vi "LSI218Data_initialize.vi"(4 "LSI218Settings(A-F)":T2(array[cluster])=[{"LSIName"="LSI218A", "Labels"=["N.C.", "N.C.", "N.C.", "N.C.", "N.C.", "N.C.", "N.C.", "N.C."], "SensorLocations"=[enum."N.C.", enum."N.C.", enum."N.C.", enum."N.C.", enum."N.C.", enum."N.C.", enum."N.C.", enum."N.C."], "Active?"=FALSE, "VISA res. name"=""}, {"LSIName"="LSI218B", "Labels"=["N.C.", "N.C.", "N.C.", "N.C.", "N.C.", "N.C.", "N.C.", "N.C."], "SensorLocations"=[enum."N.C.", enum."N.C.", enum."N.C.", enum."N.C.", enum."N.C.", enum."N.C.", enum."N.C.", enum."N.C."], "Active?"=FALSE, "VISA res. name"=""}, {"LSIName"="LSI218C", "Labels"=["N.C.", "N.C.", "N.C.", "N.C.", "N.C.", "N.C.", "N.C.", "N.C."], "SensorLocations"=[enum."N.C.", enum."N.C.", enum."N.C.", enum."N.C.", enum."N.C.", enum."N.C.", enum."N.C.", enum."N.C."], "Active?"=FALSE, "VISA res. name"=""}, {"LSIName"="LSI218D", "Labels"=["N.C.", "N.C.", "N.C.", "N.C.", "N.C.", "N.C.", "N.C.", "N.C."], "SensorLocations"=[enum."N.C.", enum."N.C.", enum."N.C.", enum."N.C.", enum."N.C.", enum."N.C.", enum."N.C.", enum."N.C."], "Active?"=FALSE, "VISA res. name"=""}, {"LSIName"="LSI218E", "Labels"=["N.C.", "N.C.", "N.C.", "N.C.", "N.C.", "N.C.", "N.C.", "N.C."], "SensorLocations"=[enum."N.C.", enum."N.C.", enum."N.C.", enum."N.C.", enum."N.C.", enum."N.C.", enum."N.C.", enum."N.C."], "Active?"=FALSE, "VISA res. name"=""}, {"LSIName"="LSI218F", "Labels"=["N.C.", "N.C.", "N.C.", "N.C.", "N.C.", "N.C.", "N.C.", "N.C."], "SensorLocations"=[enum."N.C.", enum."N.C.", enum."N.C.", enum."N.C.", enum."N.C.", enum."N.C.", enum."N.C.", enum."N.C."], "Active?"=FALSE, "VISA res. name"=""}], 5 "FileFormat":string, 7 "base path":path, 8 "error in (no error)":errorcluster, 9 "InstName":string, 10 "RunIdentifier":string, 11 "LSI218Data in":refnum<class "LSI218Data.lvclass">) -> (0 "error out":errorcluster, 1 "Status":T1(ring), 2 "AllLabels":string[](array[string]), 3 "LSI218Data out":refnum<class "LSI218Data.lvclass">)   [LabVIEW 2020, in "LSI218Data.lvclass"]
uses:
  LSI218Data.lvclass
  LSI218Data.lvclass/LSI218Data.ctl
  istr.lib/Lake Shore Cryotronics 218/Lake Shore Cryotronics 218.lvlib
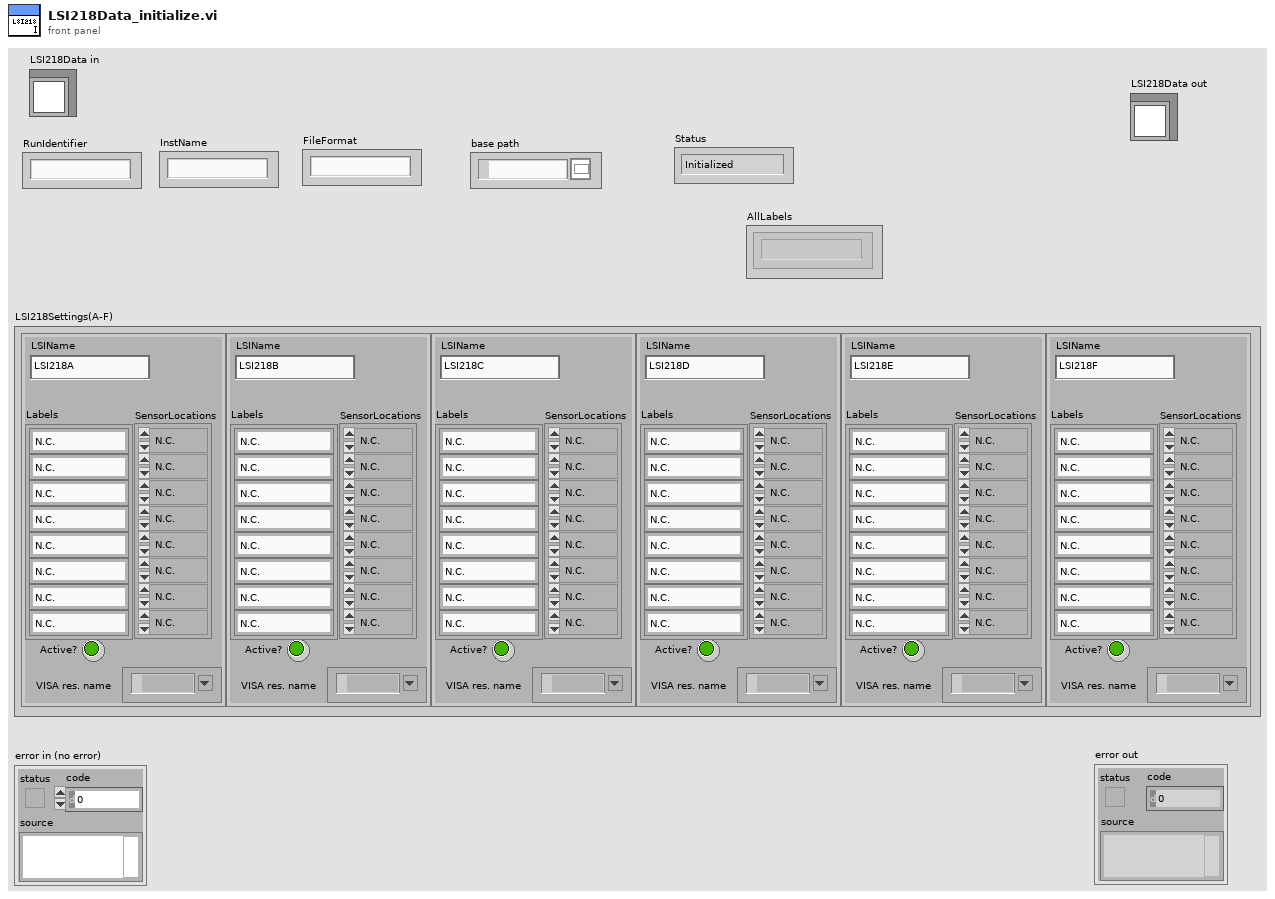
[diagram p1: front panel]
types:
  T1 = enum16{"Initialized", "Ready", "Measuring", "Terminated"}
  T2 = cluster{"LSIName":string, "Labels":string[], "SensorLocations":enum16{"N.C.", "T3He1-1", "T3He1-2", "T3He1-3", "T3He1-4", "T3He2-1", "T3He2-2", "T3He3", "T3He4", "T3He5", "T3He6-1", "T3He6-2", "T3He7-1", "T3He7-2", "T3He8", "T3He9", "T3He10", "T4He1", "T4He2-1", "T4He2-2", "T4He3-1", "T4He3-2", "T4He3-3", "T4He3-4", "T4He4", "T4He5", "T4He6", "T4He7", "T4He8", "T4He9", "T4He10", "T1K1", "T1K2", "T1K3-1", "T1K3-2", "T1K4", "T1K5", "T1K6", "TIP1", "TIP2", "TIP3", "TIP4", "TIP5", "TIP6", "TIP7", "TTH1", "TTH2", "TTH3", "TTH4"}[], "Active?":bool, "VISA res. name":refnum<visa-resource-name>}[]
  T3 = enum16{"open", "replace", "create", "open or create", "replace or create", "replace or create with confirmation"}
  T4 = cluster{"LSIName":string, "Labels":string[], "SensorLocations":enum16{"N.C.", "T3He1-1", "T3He1-2", "T3He1-3", "T3He1-4", "T3He2-1", "T3He2-2", "T3He3", "T3He4", "T3He5", "T3He6-1", "T3He6-2", "T3He7-1", "T3He7-2", "T3He8", "T3He9", "T3He10", "T4He1", "T4He2-1", "T4He2-2", "T4He3-1", "T4He3-2", "T4He3-3", "T4He3-4", "T4He4", "T4He5", "T4He6", "T4He7", "T4He8", "T4He9", "T4He10", "T1K1", "T1K2", "T1K3-1", "T1K3-2", "T1K4", "T1K5", "T1K6", "TIP1", "TIP2", "TIP3", "TIP4", "TIP5", "TIP6", "TIP7", "TTH1", "TTH2", "TTH3", "TTH4"}[], "Active?":bool, "VISA res. name":refnum<visa-resource-name>}
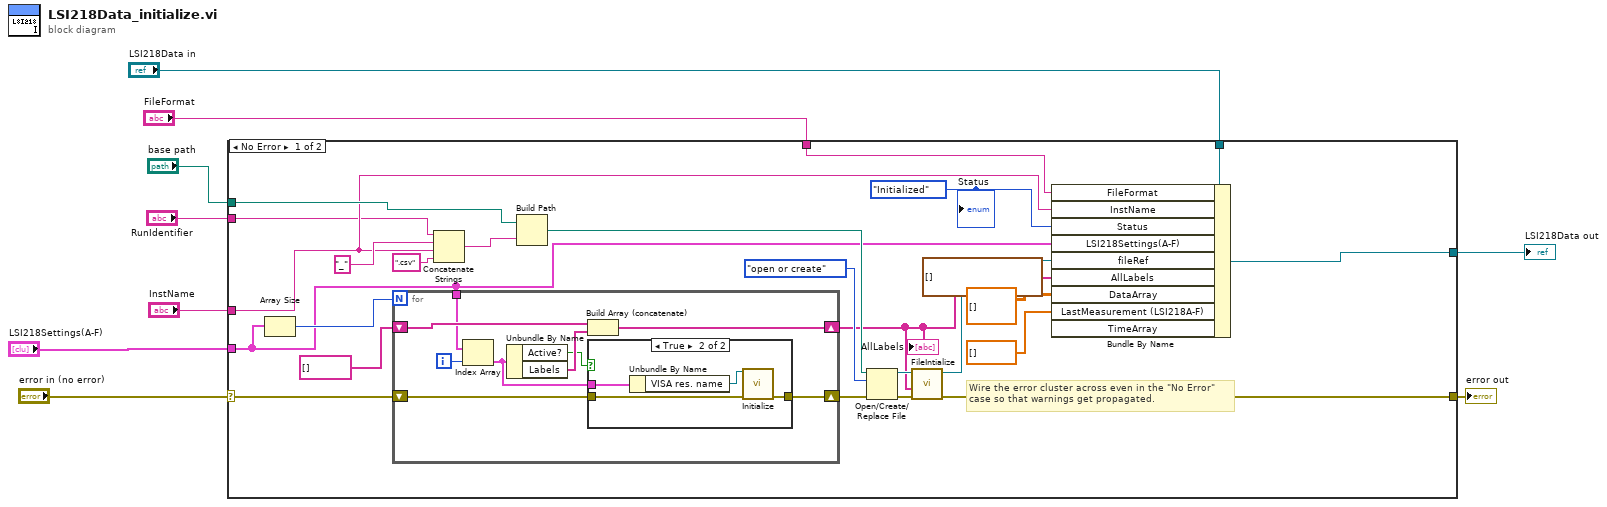
[diagram p0: block diagram]
diagram:
  n1 = case shown="No Error" "error in (no error)" {
    selector: "error in (no error)" -> [w17 w50]
    tunnel: [w16 w50] -> w8
    tunnel: [w33 w49] -> w1
    tunnel: "LSI218Settings(A-F)" -> [w12 _]
    tunnel: "RunIdentifier" -> [w10 _]
    tunnel: "InstName" -> [w18 _]
    tunnel: "base path" -> [w30 _]
    tunnel: "FileFormat" -> [w14 _]
    tunnel: "LSI218Data in" -> [w13 w49]
    frame No Error {
      w32 = T1."Initialized" ("Status")
      # "Wire the error cluster across even in the \"No Error\"\ncase so that warnings get propagated."
      n2 = Array Size(array=w12) -> (size(s)=w34:i32)
      n3 = for {
        N: w34 -> [_]
        shift-right: [w42] -> w25
        shift-left: w17 -> [w41]
        shift-right: [w40] -> w15
        shift-left: string[] [] -> [w39]
        tunnel: w12 -> [w38]
        i -> [w43]
        n4 = Index Array(array=w38, index=w43) -> (element=w35:T4)
        n5 = Unbundle By Name(w35) -> ("Active?"=w36:bool, "Labels"=w37:string[])
        n6 = Build Array (concatenate)(w39, w37) -> (w40:string[])
        n7 = case shown="True" w36 {
          tunnel: [w44 w48] -> w42
          tunnel: w41 -> [w44 w47]
          tunnel: w35 -> [_ w46]
          frame False {
          }
          frame True {
            n8 = Unbundle By Name(w46) -> ("VISA res. name"=w45:refnum<visa-resource-name>)
            n9 = call "Initialize.vi"("VISA resource name"=w45, "error in (no error)"=w47) -> ("error out"=w48:errorcluster)  [unwired: 12 in, 1 out]
          }
        }
      }
      "AllLabels" <- w15
      n10 = Concatenate Strings(w10, "_" ("string"), w18, ".csv" ("string")) -> (w26:string)
      n11 = Build Path(base path=w30, name or relative path=w26) -> (appended path=w28:path)
      n12 = Open/Create/Replace File(file path (use dialog)=w28, error in=w25, operation (0:open)=T3."open or create") -> (refnum out=w22:refnum<file>, error out=w24:errorcluster)  [unwired: 3 in, 1 out]
      n13 = call "FileIntialize.vi"("Error In"=w24, "Labels"=w15, "refnum in"=w22) -> ("Error Out"=w16:errorcluster, "File Refnum"=w21:refnum<file>)  [unwired: 7 in]
      n14 = Bundle By Name(cluster=w13, "FileFormat"=w14, "InstName"=w18, "Status"=w32, "LSI218Settings(A-F)"=w12, "fileRef"=w21, "AllLabels"=w15, "DataArray"=dbl[][] [], "LastMeasurement (LSI218A-F)"=dbl[] [], "TimeArray"=timestamp[] []) -> (w33:refnum<class "LSI218Data.lvclass">)
      "Status" <- w32
    }
    frame Error {
    }
  }
  "error out" <- w8
  "LSI218Data out" <- w1
